vi "Read configuration.vi"(8 "error in":errorcluster, 11 "tag select module editor node in":refnum<class "Table Test Editor Node.lvclass">) -> (0 "error out":errorcluster, 2 "configuration":refnum<class "NISE_CEF_serializable configuration.lvclass">, 3 "tag select module editor node out":refnum<class "Table Test Editor Node.lvclass">)   [LabVIEW 2013, in "Table Test Editor Node.lvclass"]
uses:
  Table Test Editor Node.lvclass
  <vilib>/NI/Configuration Framework/serializable configuration/NISE_CEF_serializable configuration.lvclass
  Table Test Editor Node.lvclass/Table Test Editor Node.ctl
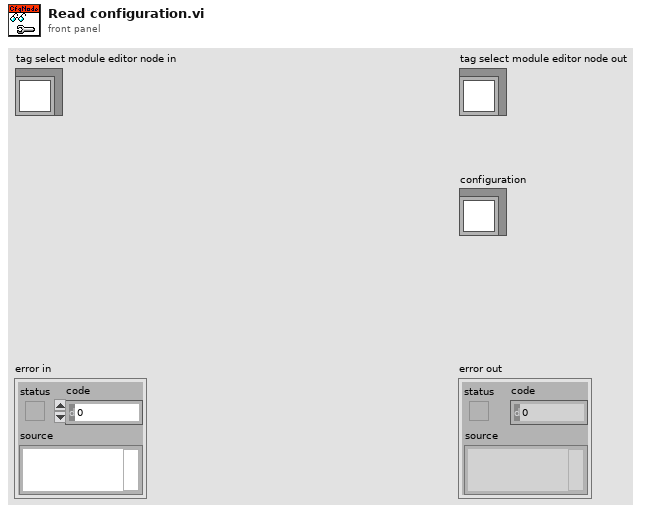
[diagram p1: front panel]
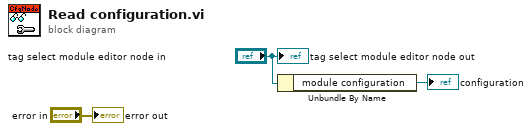
[diagram p0: block diagram]
diagram:
  n1 = Unbundle By Name("tag select module editor node in") -> ("module configuration"=→"configuration":refnum<class "Table Test configuration.lvclass">)
  "error out" <- "error in"
  "tag select module editor node out" <- "tag select module editor node in"
